vi "ID Query.vi"(8 "error in":errorcluster, 11 "VISA resource name":refnum<visa-resource-name>) -> (0 "error out":errorcluster, 1 "Serial Number":i32, 2 "Options":string, 3 "VISA resource name out":refnum<visa-resource-name>, 4 "Firmware Revision":string, 5 "Model Name":string)   [LabVIEW 2017, in "Andeen-Hagerling 2700.lvlib"]
uses:
  Andeen-Hagerling 2700.lvlib
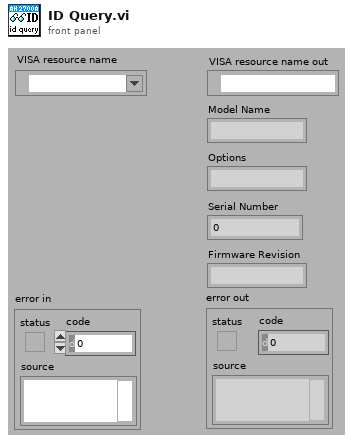
[diagram p1: front panel]
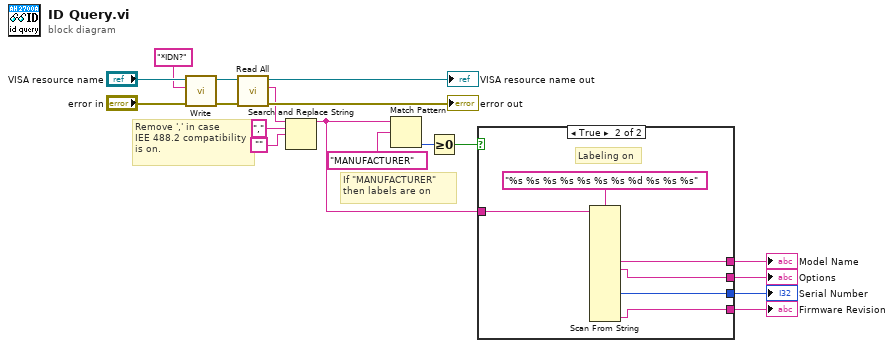
[diagram p0: block diagram]
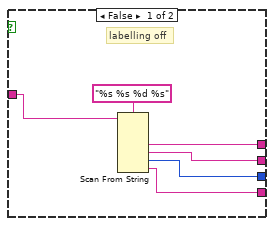
[diagram p2: hidden frame]
diagram:
  # "Remove ',' in case\nIEE 488.2 compatibility\nis on."
  # "If \"MANUFACTURER\"\nthen labels are on"
  n1 = call "Write.vi"("error in"="error in", "command"="*IDN?", "VISA resource name"="VISA resource name") -> ("error out"=w15:errorcluster, "VISA resource name out"=w14:refnum<visa-resource-name>)  [unwired: 7 in]
  n2 = call "Read All.vi"("error in"=w15, "VISA resource name"=w14) -> ("error out"=→"error out":errorcluster, "Message"=w11:string, "VISA resource name out"=→"VISA resource name out":refnum<visa-resource-name>)  [unwired: 6 in, 1 out]
  n3 = Search and Replace String(input string=w11, search string=",", replace string="") -> (result string=w6:string)  [unwired: 5 in, 3 out]
  n4 = Match Pattern(string=w6, regular expression="MANUFACTURER" ("y")) -> (offset past match=w7:i32)  [unwired: 1 in, 3 out]
  n5 = Greater Or Equal To 0?(x=w7) -> (x >= 0?=w5:bool)
  n6 = case shown="True" w5 {
    tunnel: w6 -> [w19 w30]
    tunnel: [w23 w28] -> w4
    tunnel: [w22 w27] -> w3
    tunnel: [w21 w26] -> w2
    tunnel: [w20 w25] -> w1
    frame False {
      # "labelling off"
      n7 = Scan From String(format string="%s %s %d %s", input string=w19) -> (output 1=w23:string, output 2=w22:string, output 3=w21:i32, output 4=w20:string)  [unwired: 6 in, 3 out]
    }
    frame True {
      # "Labeling on"
      n8 = Scan From String(format string="%s %s %s %s %s %s %s %d %s %s %s", input string=w30) -> (output 4=w28:string, output 5=w27:string, output 8=w26:i32, output 11=w25:string)  [unwired: 20 in, 3 out]
    }
  }
  "Model Name" <- w4
  "Options" <- w3
  "Serial Number" <- w2
  "Firmware Revision" <- w1
